vi "Image Measure.vi"() -> ()   [LabVIEW 2016]
panel:
  out "Line length":dbl format="%#_6pm"
  in  "Reference length":dbl=0.005 format="%#_6pm"
  in  "Calibration":dbl=1.5681962050709619e-06 format="%#_6pm/pixel"
  in  "Calibrate Button":bool
  out "Line pixel length":dbl
  out "Line":T1 {"Start X" scale=0.0..1024.0; "End X" scale=0.0..1024.0}
  out "ROI":T2
  out "Tool":i32(ring) items=["None", "Selection Tool", "Point Tool", "Line Tool", "Rectangle Tool", "Oval Tool", "Polygon Tool", "ClosedFreehandTool", "Annulus Tool", "Rotated Rectangle Tool", "Zoom Tool", "Pan Tool", "Polyline Tool", "Freehand Tool"]
  out "Type":i32(ring) items=["No Event"=0, "Click Event"=1, "Draw Event"=2, "Size Event"=4, "Scroll Event"=5, "Double Click Event"=8]
  in  "Stop Button":bool
  in  "Image 1 path":path
  out "Image":T3(plugin-control)
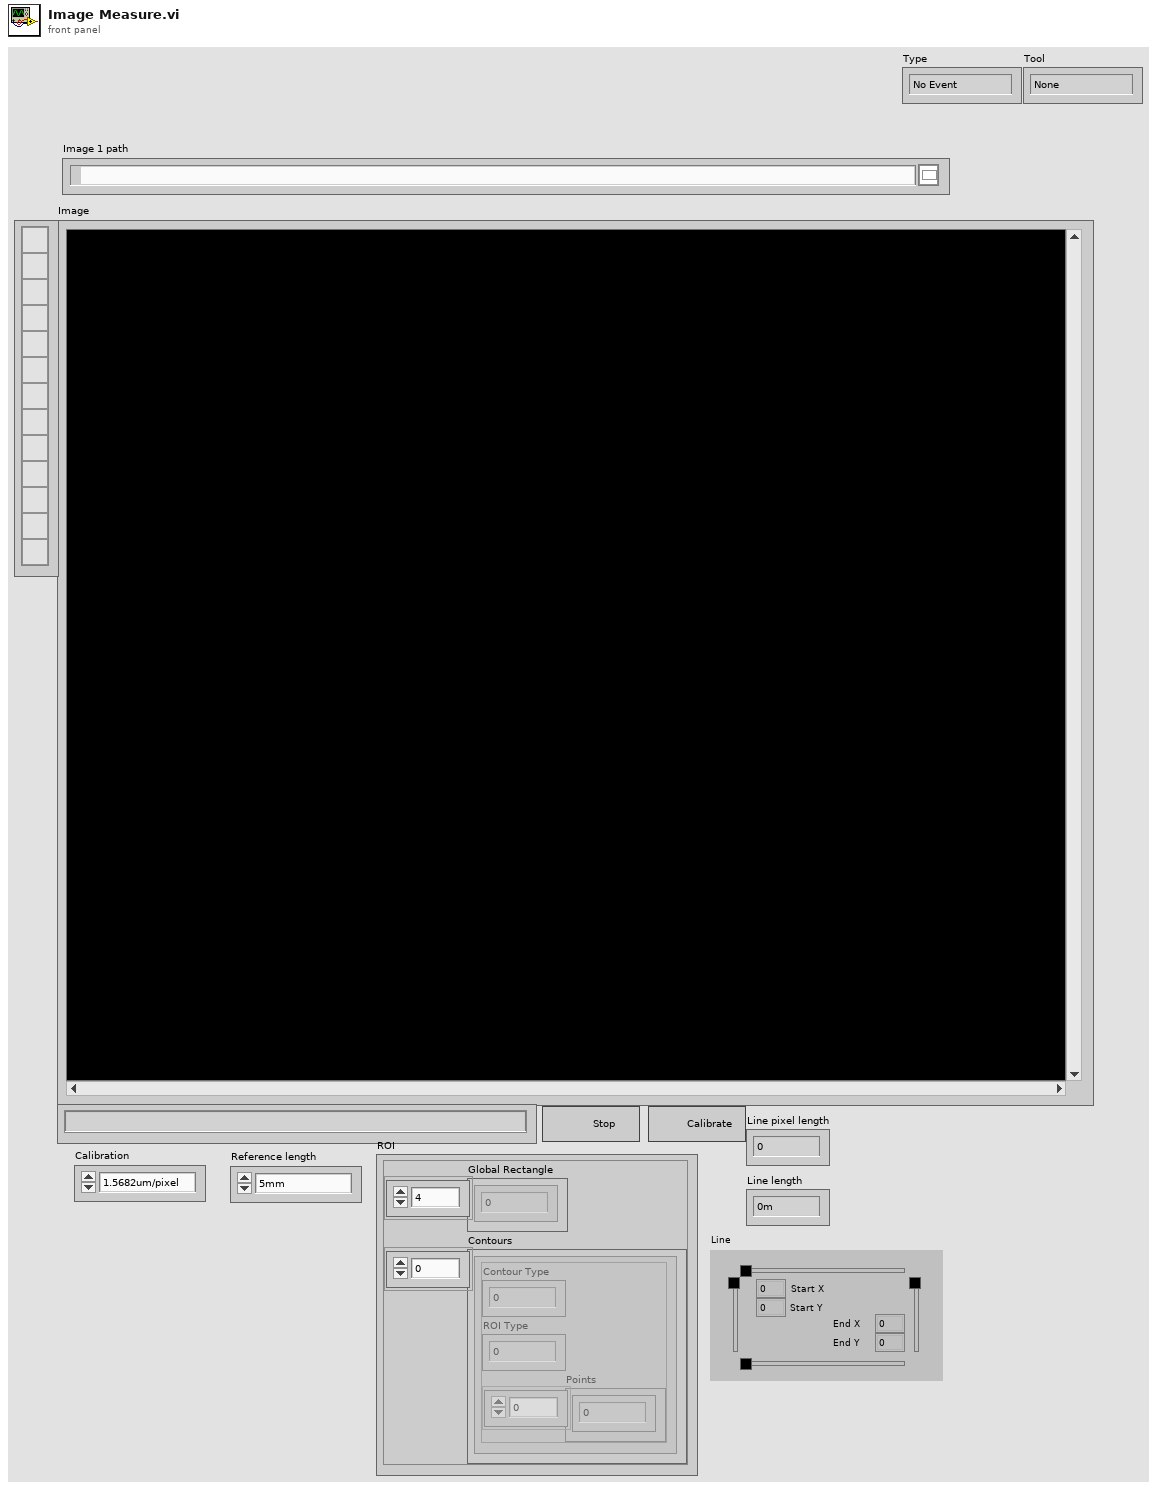
[diagram p1: front panel]
types:
  T1 = typedef "IMAQ Line" = cluster{"Start X":i32, "Start Y":i32, "End X":i32, "End Y":i32}
  T2 = cluster{"Global Rectangle":i32[], "Contours":cluster{"Contour Type":u32, "ROI Type":u32, "Points":i32[]}[]}
  T3 = typedef "IMAQ Image.ctl" = refnum<image>
  T4 = typedef "Image Type" = u32
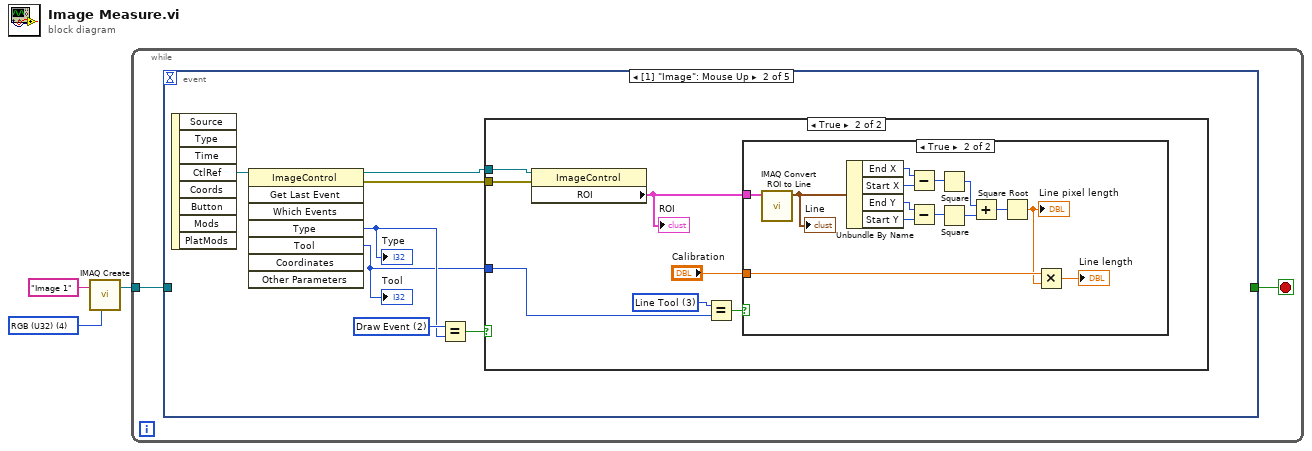
[diagram p0: block diagram]
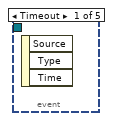
[diagram p2: hidden frame]
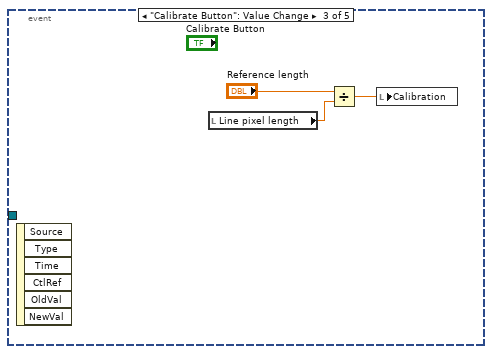
[diagram p5: hidden frame]
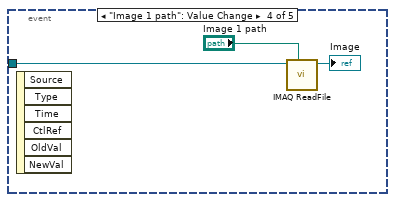
[diagram p6: hidden frame]
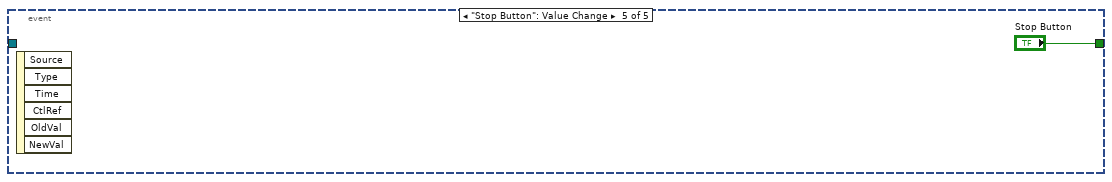
[diagram p7: hidden frame]
diagram:
  w2 = T4 4 items=["Grayscale (U8)", "Grayscale (I16)", "Grayscale (SGL)", "Complex (CSG)", "RGB (U32)", "HSL (U32)", "RGB (U64)", "Grayscale (U16)"] ("Image Type")
  n1 = call "IMAQ Create"("Image Name"="Image 1", "Image Type"=w2) -> ("New Image"=w1:T3)  [unwired: 3 in, 1 out]
  n2 = while {
    tunnel: w1 -> [w4]
    stop <- w5 stop-if-true
    n3 = event shown="[1] \"Image\": Mouse Up" {
      selector: _ -> [_ _ _ _ _]
      dyn-events: _ -> [_ _ _ _ _]
      timeout: _ -> [_ _ _ _ _]
      tunnel: [_ _ _ _ "Stop Button"] -> w5
      tunnel: w4 -> [_ _ _ w38 _]
      event Timeout {
        n4 = event-data() -> ()  [unwired: 1 in, 3 out]
      }
      event "Image": Mouse Up {
        w11 = 2 items=["No Event"=0, "Click Event"=1, "Draw Event"=2, "Size Event"=4, "Scroll Event"=5, "Double Click Event"=8] ("Type")
        n5 = event-data() -> ("CtlRef"=w12:refnum<vi>)  [unwired: 1 in, 7 out]
        n6 = invoke class="ImageControl" method="Get Last Event"(reference=w12) -> (reference out=w9:refnum<vi>, error out=w8:errorcluster, "Type"=w10:i32, "Tool"=w7:i32)  [unwired: 7 in, 4 out]
        "Type" <- w10
        "Tool" <- w7
        n7 = Equal?(x=w11, y=w10) -> (x = y?=w6:bool)
        n8 = case shown="True" w6 {
          tunnel: w9 -> [_ w19]
          tunnel: w8 -> [_ w18]
          tunnel: w7 -> [_ w14]
          frame False {
          }
          frame True {
            w15 = 3 items=["None", "Selection Tool", "Point Tool", "Line Tool", "Rectangle Tool", "Oval Tool", "Polygon Tool", "ClosedFreehandTool", "Annulus Tool", "Rotated Rectangle Tool", "Zoom Tool", "Pan Tool", "Polyline Tool", "Freehand Tool"] ("Tool")
            n9 = property class="ImageControl"(reference=w19, error in=w18) -> ("ROI"=w17:T2)  [unwired: 2 out]
            "ROI" <- w17
            n10 = Equal?(x=w15, y=w14) -> (x = y?=w13:bool)
            n11 = case shown="True" w13 {
              tunnel: w17 -> [_ w33]
              tunnel: "Calibration" -> [_ w22]
              frame False {
              }
              frame True {
                n12 = call "IMAQ Convert ROI to Line"("ROI Descriptor"=w33) -> ("Line"=w32:T1)  [unwired: 8 in, 1 out]
                "Line" <- w32
                n13 = Unbundle By Name(w32) -> ("End X"=w31:i32, "Start X"=w30:i32, "End Y"=w29:i32, "Start Y"=w28:i32)
                n14 = Subtract(x=w31, y=w30) -> (x-y=w27:i32)
                n15 = Subtract(x=w29, y=w28) -> (x-y=w26:i32)
                n16 = Square(x=w27) -> (x^2=w25:i32)
                n17 = Square(x=w26) -> (x^2=w24:i32)
                n18 = Add(x=w25, y=w24) -> (x+y=w23:i32)
                n19 = Square Root(x=w23) -> (sqrt(x)=w21:dbl)
                "Line pixel length" <- w21
                n20 = Multiply(x=w22, y=w21) -> (x*y=→"Line length":dbl)
              }
            }
          }
        }
      }
      event "Calibrate Button": Value Change {
        n21 = event-data() -> ()  [unwired: 1 in, 6 out]
        n22 = local read "Line pixel length"() -> (w34:dbl)
        n23 = Divide(x="Reference length", y=w34) -> (x/y=w35:dbl)
        n24 = local write "Calibration"(w35) -> ()
      }
      event "Image 1 path": Value Change {
        n25 = event-data() -> ()  [unwired: 1 in, 6 out]
        n26 = call "IMAQ ReadFile"("File Path"="Image 1 path", "Image"=w38) -> ("Image Out"=→"Image":T3)  [unwired: 5 in, 4 out]
      }
      event "Stop Button": Value Change {
        n27 = event-data() -> ()  [unwired: 1 in, 6 out]
      }
    }
  }
